vi "FGV.vi"(7 "Action":T1, 8 "error in (no error)":errorcluster, 9 "IAmGLF Return Notifier":refnum<notifier>, 10 "IAmGLF To Create DVR":refnum<class "IAmGLF.lvclass">, 11 "IAmEngine":refnum<class "IAmEngine.lvclass">) -> (0 "error out":errorcluster)   [LabVIEW 2024, in "GLF.lvlib" / "DVRHandler.lvlib"]
uses:
  DVRHandler.lvlib
  IAmEngine/IAmEngine.lvclass
  IAmGLF/IAmGLF.lvclass
  Action--enum.ctl
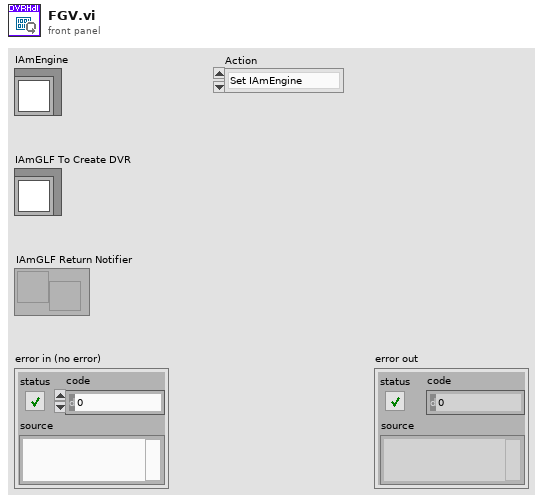
[diagram p1: front panel]
types:
  T1 = typedef "GLF.lvlib/DVRHandler.lvlib/Action--enum.ctl" = enum16{"Set IAmEngine", "Create DVR"}
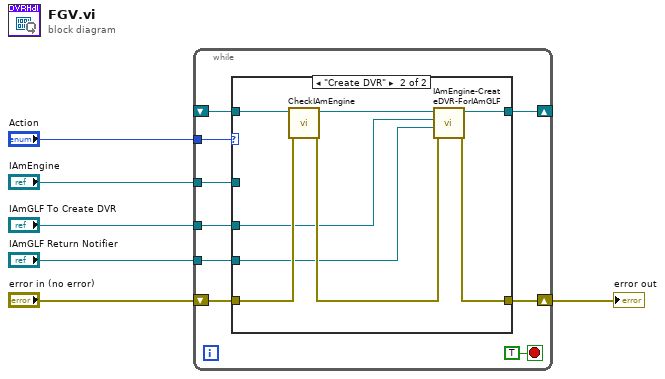
[diagram p0: block diagram]
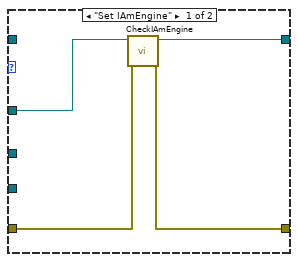
[diagram p2: hidden frame]
diagram:
  n1 = while {
    tunnel: "IAmEngine" -> [w15]
    tunnel: "IAmGLF To Create DVR" -> [w13]
    tunnel: "IAmGLF Return Notifier" -> [w12]
    tunnel: "Action" -> [w10]
    shift-right: [w11] -> w2
    shift-left: "error in (no error)" -> [w14]
    shift-right: [w8] -> _
    shift-left: _ -> [w7]
    stop <- TRUE stop-if-true
    n2 = case shown="\"Create DVR\"" w10 {
      tunnel: w15 -> [w19 _]
      tunnel: w14 -> [w17 w26]
      tunnel: w13 -> [_ w25]
      tunnel: w12 -> [_ w24]
      tunnel: [w16 w23] -> w11
      tunnel: [w18 w21] -> w8
      tunnel: w7 -> [_ w22]
      frame "Set IAmEngine" {
        n3 = call "CheckIAmEngine.vi"("error in (no error)"=w17, "IAmEngine In"=w19) -> ("error out"=w16:errorcluster, "IAmEngine Out"=w18:refnum<class "IAmEngine.lvclass">)  [unwired: 8 in]
      }
      frame "Create DVR" {
        n4 = call "CheckIAmEngine.vi"("error in (no error)"=w26, "IAmEngine In"=w22) -> ("error out"=w27:errorcluster, "IAmEngine Out"=w20:refnum<class "IAmEngine.lvclass">)  [unwired: 8 in]
        n5 = call-dynamic "IAmEngine-CreateDVR-ForIAmGLF.vi"("error in (no error)"=w27, "IAmGLF Return Notifier"=w24, "IAmGLF To Create DVR"=w25, "IAmEngine in"=w20) -> ("error out"=w23:errorcluster, "IAmEngine out"=w21:refnum<class "IAmEngine.lvclass">)  [unwired: 6 in]
      }
    }
  }
  "error out" <- w2
